vi "Metronome.vi"() -> ()   [LabVIEW 2015]
panel:
  in  "stop":bool
  in  "Beats Per Minute":dbl
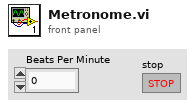
[diagram p1: front panel]
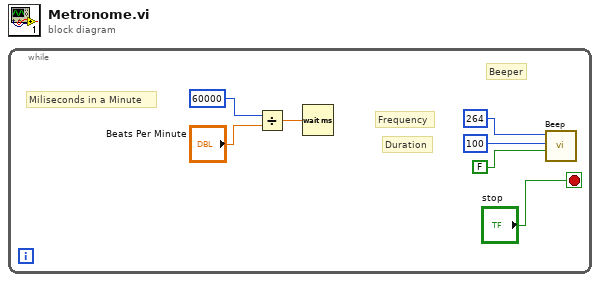
[diagram p0: block diagram]
diagram:
  n1 = while {
    stop <- "stop" stop-if-true
    # "Beeper"
    # "Duration"
    # "Frequency"
    # "Miliseconds in a Minute"
    n2 = Divide(x=60000, y="Beats Per Minute") -> (x/y=w2:dbl)
    n3 = Wait (ms)(milliseconds to wait=w2) -> ()  [unwired: 1 out]
    n4 = call <vilib>:"Beep.vi"("use system alert? (T)"=FALSE, "duration (msec)"=u32 100, "frequency (Hz)"=u32 264) -> ()  [unwired: 9 in]
  }
